vi "KDC101_Close.vi"(8 "error in (no error)":errorcluster caption="entrée d'erreur (pas d'erreur)", 11 "KCubeDCServoRefIn":refnum<k24>) -> (0 "error out":errorcluster caption="sortie d'erreur", 1 "Connected":bool, 3 "KCubeDCServoRef":refnum<k24>)   [LabVIEW 2019]
doc: "Utilisez ce modèle pour construire un VI à utiliser en tant que sous-VI."
uses:
  C:/Program Files (x86)/National Instruments/LabVIEW 2019/user.lib/ThorKDC101/Kinesis_with_LabVIEW_Examples_LV12 - v3/ThorLabs.MotionControl.KCube.DCServoCLI.dll
  Kinesis_with_LabVIEW_Examples_LV12 - v3/ThorLabs.MotionControl.KCube.DCServoCLI.dll
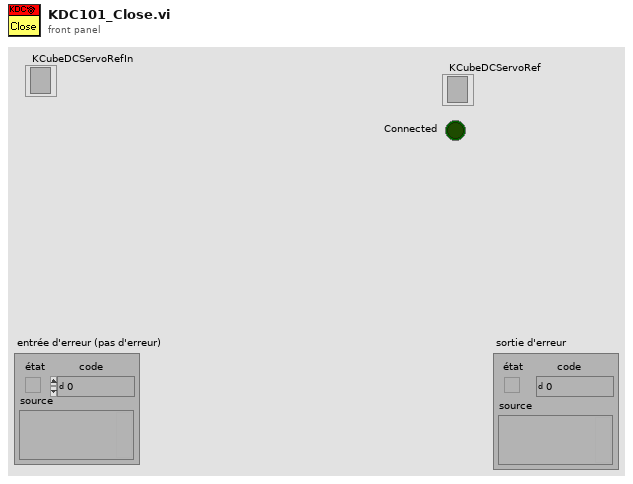
[diagram p1: front panel]
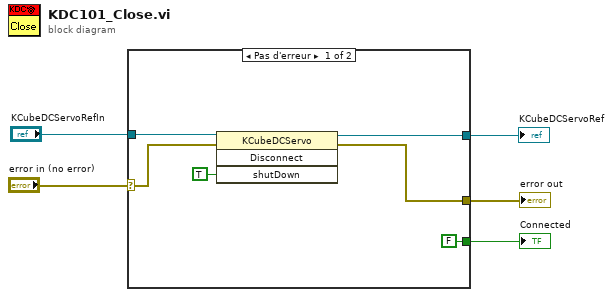
[diagram p0: block diagram]
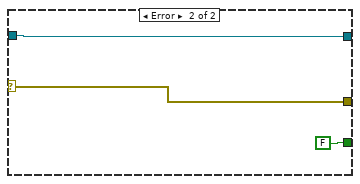
[diagram p2: hidden frame]
diagram:
  n1 = case shown="Pas d'erreur" "error in (no error)" {
    selector: "error in (no error)" -> [w10 w14]
    tunnel: [w7 w14] -> w4
    tunnel: [FALSE FALSE] -> w3
    tunnel: "KCubeDCServoRefIn" -> [w9 w12]
    tunnel: [w8 w12] -> w1
    frame No Error {
      n2 = invoke class="KCubeDCServo" method="Disconnect"(reference=w9, error in=w10, "shutDown"=TRUE) -> (reference out=w8:refnum<k24>, error out=w7:errorcluster)  [unwired: 1 in, 2 out]
    }
    frame Error {
    }
  }
  "error out" <- w4
  "KCubeDCServoRef" <- w1
  "Connected" <- w3
